vi "Clear Display.vi"(8 "error in (no error)":errorcluster, 11 "RPI.SenseHat.Actor in":refnum<class "RPI.SenseHat.Actor.lvclass">) -> (0 "error out":errorcluster, 3 "RPI.SenseHat.Actor out":refnum<class "RPI.SenseHat.Actor.lvclass">)   [LabVIEW 2020, in "RPI.SenseHat.Actor.lvlib" / "RPI.SenseHat.Actor.lvclass"]
uses:
  RPI.SenseHat.Actor.lvclass
  RPI.SenseHat.Actor.lvclass/RPI.SenseHat.Actor.ctl
  RPI.SenseHat/SenseHat/SenseHat.lvclass/SenseHat.ctl
  RPI.SenseHat/SenseHat/Get RPI.SenseHat.Display.vi
  RPI.SenseHat.Display/Classes/SenseHat.Display/RPI.SenseHat.Display.lvclass
  RPI.SenseHat/SenseHat/SenseHat.lvclass
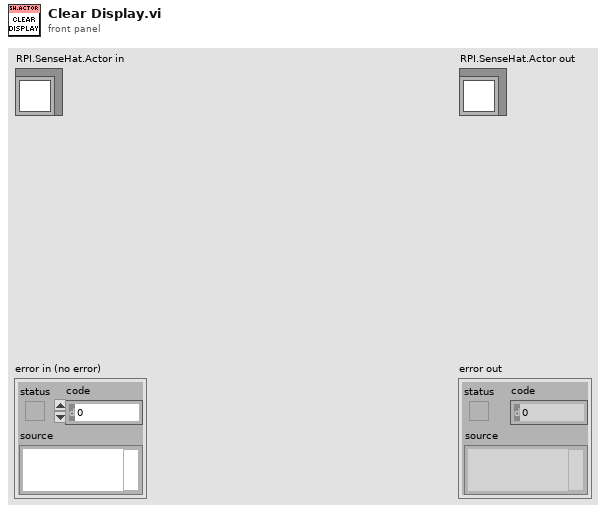
[diagram p1: front panel]
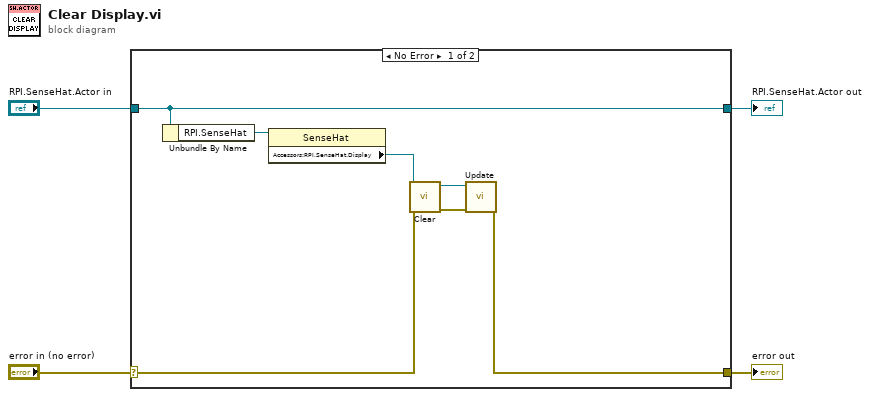
[diagram p0: block diagram]
diagram:
  n1 = case shown="No Error" "error in (no error)" {
    selector: "error in (no error)" -> [w6 w13]
    tunnel: [w5 w13] -> w3
    tunnel: [w7 w12] -> w1
    tunnel: "RPI.SenseHat.Actor in" -> [w7 w12]
    frame No Error {
      n2 = Unbundle By Name(w7) -> ("RPI.SenseHat"=w11:refnum<class "SenseHat.lvclass">)
      n3 = property class="SenseHat"(reference=w11) -> ("Accessors:RPI.SenseHat.Display"=w10:refnum<class "RPI.SenseHat.Display.lvclass">)  [unwired: 1 in, 2 out]
      n4 = call "Clear.vi"("error in (no error)"=w6, "senseHatDisplay in"=w10) -> ("error out"=w8:errorcluster, "senseHatDisplay out"=w9:refnum<class "RPI.SenseHat.Display.lvclass">)  [unwired: 8 in]
      n5 = call "Update.vi"("error in (no error)"=w8, "senseHatDisplay in"=w9) -> ("error out"=w5:errorcluster)  [unwired: 8 in, 1 out]
    }
    frame Error {
    }
  }
  "error out" <- w3
  "RPI.SenseHat.Actor out" <- w1
